vi "Nonlinear model fit example.vi"() -> ()   [LabVIEW 2009]
uses:
  <vilib>/gmath/NumericalOptimization/Nonlinear Curve Fit LM formula string.vi
  <vilib>/gmath/NI_Gmath.lvlib
panel:
  out "best fit parameters":dbl[](array[numeric])
  in  "initial parameters":dbl[](array[numeric])=[0.0, 0.0, 0.0, 0.0]
  in  "X":dbl[](array[numeric])=[1.0, 2.0, 3.0, 4.0, 5.0, 6.0]
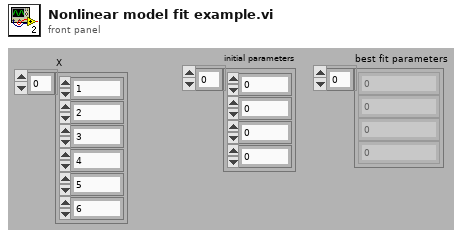
[diagram p1: front panel]
types:
  T1 = cluster{"model":string, "Parameters":string[], "x":string}
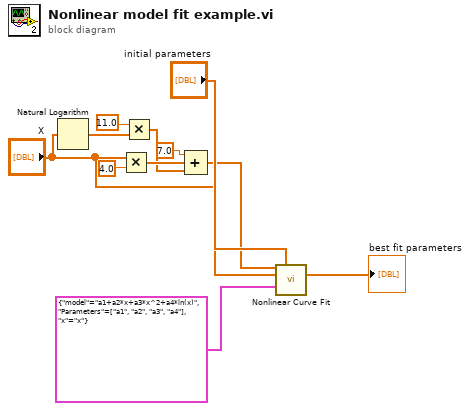
[diagram p0: block diagram]
diagram:
  n1 = Natural Logarithm(1:"X") -> (0:w6:dbl[])
  n2 = Multiply(x="X", y=4.0 ("x")) -> (x*y=w7:dbl[])
  n3 = Multiply(x=11.0, y=w6) -> (x*y=w4:dbl[])
  n4 = Compound Arithmetic op=ADD(7.0 ("x"), w7, w4) -> (w3:dbl[])
  n5 = call-poly <vilib>:"Nonlinear Curve Fit.vi"("Y"=w3, "initial parameters"="initial parameters", "X"="X", "model description"=T1 {"model"="a1+a2*x+a3*x^2+a4*ln(x)", "Parameters"=["a1", "a2", "a3", "a4"], "x"="x"}) -> ("best fit parameters"=→"best fit parameters":dbl[])  [unwired: 7 in, 4 out]
